vi "GetDigitalFilterControl.vi"(8 "Error In":errorcluster, 10 "Channel (1 or 2)":u8=1 min=1 max=2 step=1, 11 "Keithley 6482 In":refnum<visa-resource-name>) -> (0 "Error Out":errorcluster, 2 "Digital Filter Control":T1, 3 "Keithley 6482 Out":refnum<visa-resource-name>)   [LabVIEW 2012, in "Keithley-6482.lvlib"]
uses:
  Keithley-6482.lvlib
  Controls/DigitalFilterControl.ctl
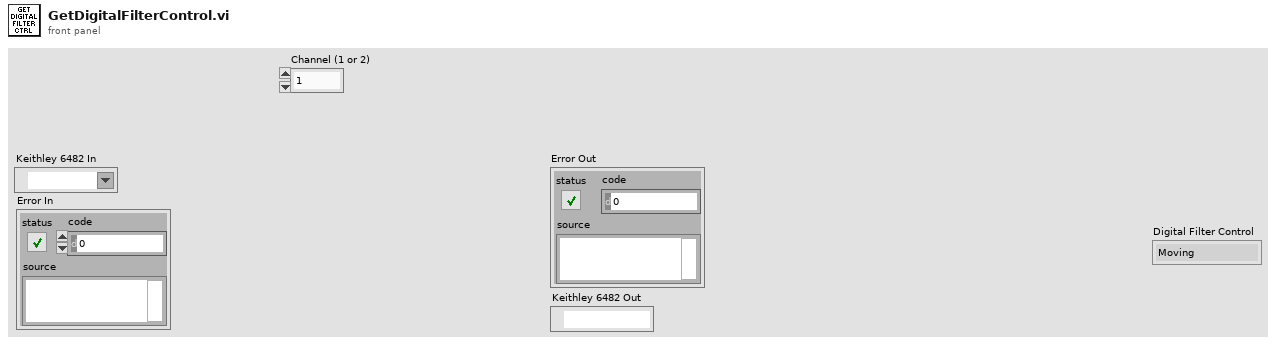
[diagram p1: front panel]
types:
  T1 = typedef "Keithley-6482.lvlib/DigitalFilterControl.ctl" = enum16{"Moving", "Repeat"}
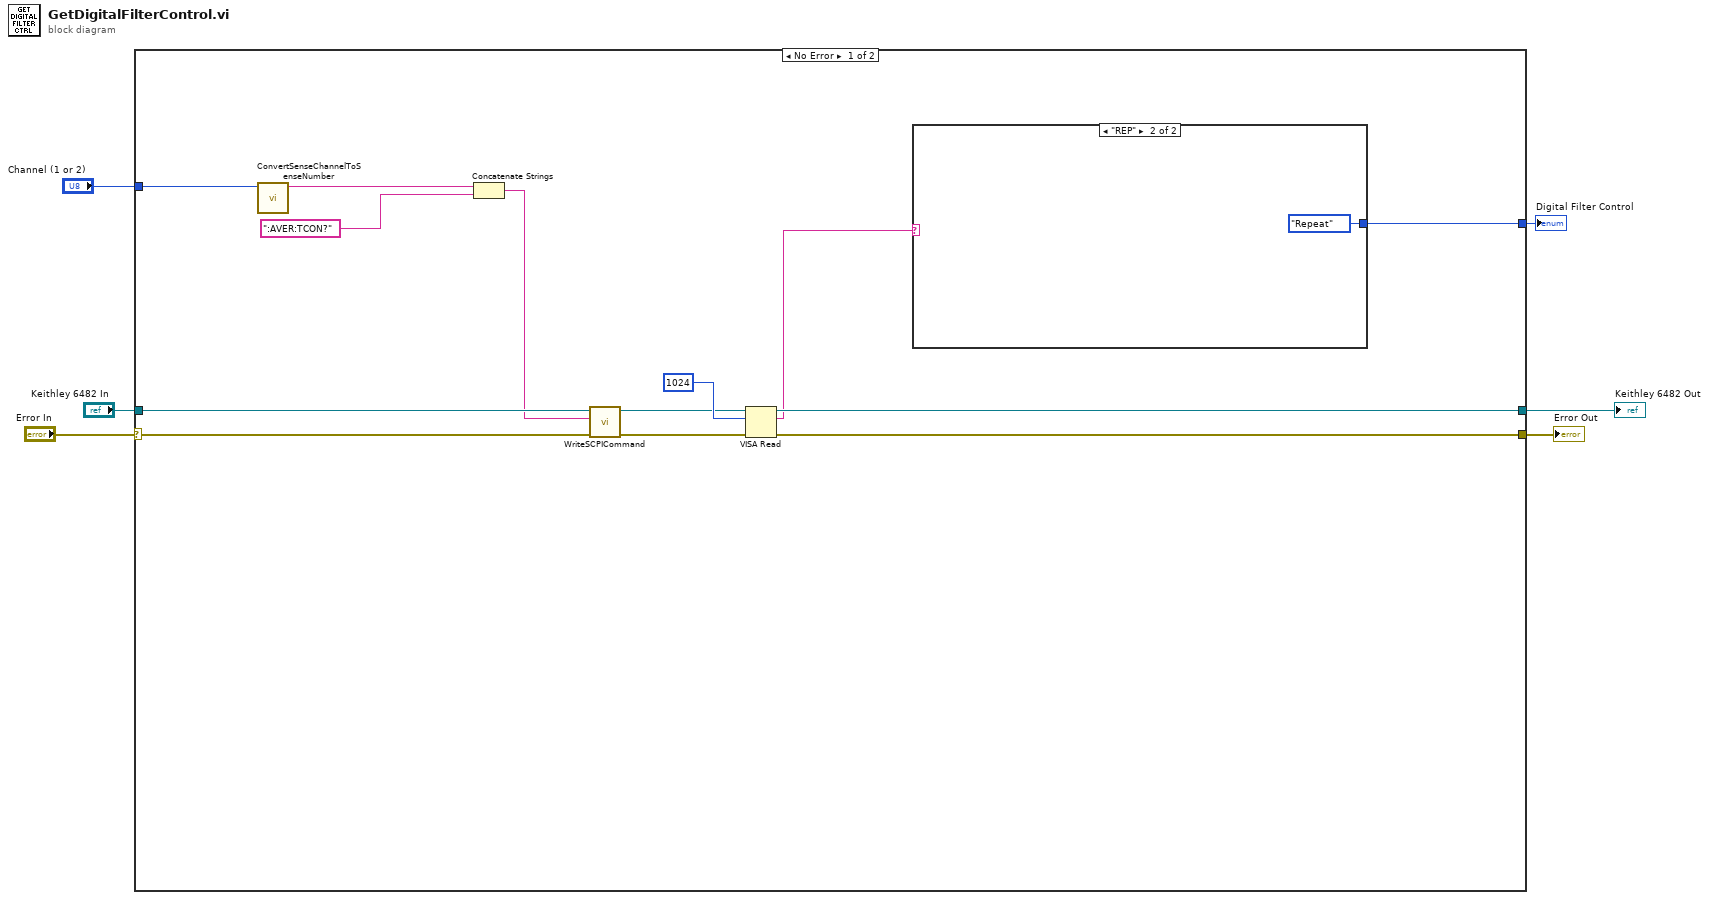
[diagram p0: block diagram]
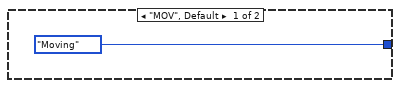
[diagram p2: hidden frame]
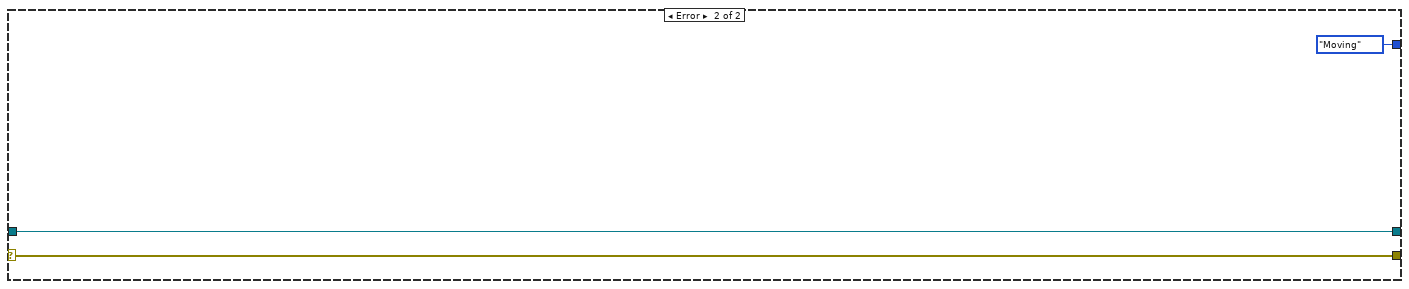
[diagram p3: hidden frame]
diagram:
  n1 = case shown="No Error" "Error In" {
    selector: "Error In" -> [w14 w23]
    tunnel: "Keithley 6482 In" -> [w13 w24]
    tunnel: [w19 w23] -> w4
    tunnel: [w18 w24] -> w3
    tunnel: "Channel (1 or 2)" -> [w12 _]
    tunnel: [w7 DigitalFilterControl."Moving" ("Filter Control")] -> w1
    frame No Error {
      n2 = call "ConvertSenseChannelToSenseNumber.vi"("Channel (1 or 2)"=w12) -> ("Sense Number"=w11:string)  [unwired: 10 in]
      n3 = Concatenate Strings(w11, ":AVER:TCON?" ("string")) -> (w9:string)
      n4 = call "WriteSCPICommand.vi"("Error In"=w14, "SCPI Command"=w9, "Keithley 6482 In"=w13) -> ("Error Out"=w15:errorcluster, "Keithley 6482 Out"=w16:refnum<visa-resource-name>)  [unwired: 7 in]
      n5 = VISA Read(VISA resource name=w16, byte count=u32 1024, error in (no error)=w15) -> (VISA resource name out=w18:refnum<visa-resource-name>, read buffer=w8:string, error out=w19:errorcluster)  [unwired: 1 out]
      n6 = case shown="\"REP\"" w8 {
        tunnel: [DigitalFilterControl."Moving" ("Filter Control") DigitalFilterControl."Repeat" ("Filter Control")] -> w7
        frame "MOV", Default {
        }
        frame "REP" {
        }
      }
    }
    frame Error {
    }
  }
  "Error Out" <- w4
  "Keithley 6482 Out" <- w3
  "Digital Filter Control" <- w1
